vi "更新批次.vi"(8 "error in (no error)":errorcluster caption="错误输入", 11 "型号":string) -> (0 "error out":errorcluster caption="错误输出")   [LabVIEW 2018]
uses:
  <vilib>/addons/database/Connection.llb/DB Tools Open Connec (String).vi
  <vilib>/addons/database/Connection.llb/Conn Execute.vi
  <vilib>/addons/database/Recordset.llb/Rec Fetch Recordset Data (R).vi
  <vilib>/addons/database/Recordset.llb/Rec Destroy - Connection.vi
  <vilib>/addons/database/NI_Database_API.lvlib
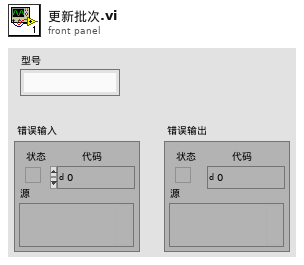
[diagram p1: front panel]
types:
  T1 = typedef "NI_Database_API.lvlib/Conn ObjectReference.ctl" = refnum<k1>
  T2 = typedef "NI_Database_API.lvlib/Rec ObjectReference.ctl" = refnum<k1>
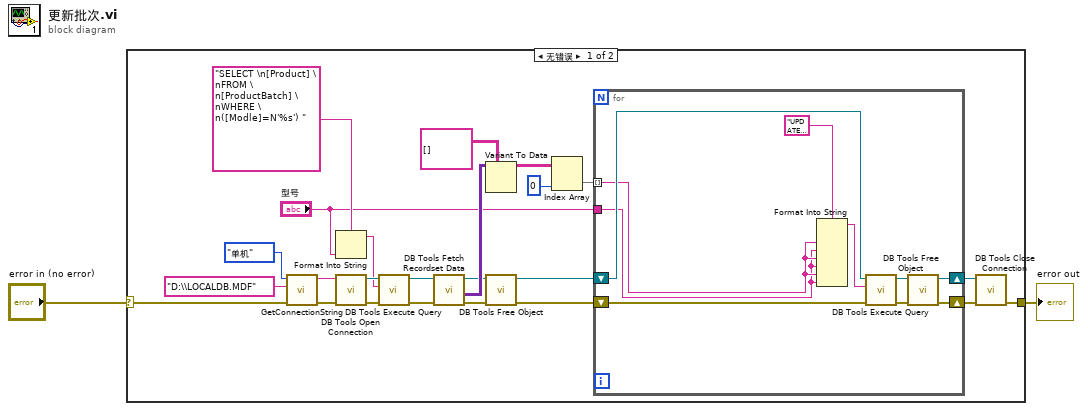
[diagram p0: block diagram]
diagram:
  n1 = case shown="无错误" "error in (no error)" {
    selector: "error in (no error)" -> [w6 w37]
    tunnel: [w19 w37] -> w1
    frame No Error {
      n2 = call "GetConnectionString.vi"("error in (no error)"=w6, "Database Name"="D:\\LOCALDB.MDF", "连接模式"=enum16{"单机", "联网"}."单机") -> ("error out"=w25:errorcluster, "连接字符串"=w24:string)  [unwired: 3 in]
      n3 = Format Into String(format string="SELECT \n[Product] \nFROM \n[ProductBatch] \nWHERE \n([Modle]=N'%s') " ("SQL query"), "型号") -> (resulting string=w4:string)  [unwired: 2 in, 1 out]
      n4 = call-poly <vilib>:"DB Tools Open Connection.vi"("error in (no error)"=w25, "connection information"=w24) -> ("error out"=w23:errorcluster, "connection reference"=w22:T1)  [unwired: 6 in]
      n5 = call-poly <vilib>:"DB Tools Execute Query.vi"("error in (no error)"=w23, "SQL query"=w4, "connection reference"=w22) -> ("error out"=w18:errorcluster, "recordset reference"=w17:T2)  [unwired: 5 in]
      n6 = call-poly <vilib>:"DB Tools Fetch Recordset Data.vi"("error in (no error)"=w18, "recordset reference"=w17) -> ("error out"=w11:errorcluster, "recordset data"=w16:variant[][], "recordset reference out"=w12:T2)  [unwired: 3 in]
      n7 = Variant To Data(type=string[][] [], Variant=w16) -> (data=w14:string[][])  [unwired: 1 in, 1 out]
      n8 = call-poly <vilib>:"DB Tools Free Object.vi"("error in (no error)"=w11, "recordset reference"=w12) -> ("error out"=w9:errorcluster, "connection reference"=w10:T1)  [unwired: 8 in]
      n9 = Index Array(array=w14, index (col)=0 ("禁用的索引 (列)")) -> (element=w8:string[])  [unwired: 1 in]
      n10 = for {
        shift-right: [w35] -> w20
        shift-left: w10 -> [w31]
        shift-right: [w36] -> w21
        shift-left: w9 -> [w30]
        tunnel: w8 -> [w28] mode=indexing
        tunnel: "型号" -> [w27]
        n11 = Format Into String(format string="UPDATE [ProductBatch] \nSET [Used]=(SELECT \n[Used] \nFROM \n[ProductBatch] \nWHERE \n[Product] =N'%s' AND \n[Modle]=N'%s')+(SELECT \n[Time] \nFROM \n[ProductBatch] \nWHERE \n[Product] =N'%s' AND \n[Modle]=N'%s') \nWHERE ([Product] =N'%s' \nAND [Modle]=N'%s') " ("格式字符串"), w28, w27, w28, w27, w28, w27) -> (resulting string=w29:string)  [unwired: 2 in, 1 out]
        n12 = call-poly <vilib>:"DB Tools Execute Query.vi"("error in (no error)"=w30, "SQL query"=w29, "connection reference"=w31) -> ("error out"=w32:errorcluster, "recordset reference"=w33:T2)  [unwired: 5 in]
        n13 = call-poly <vilib>:"DB Tools Free Object.vi"("error in (no error)"=w32, "recordset reference"=w33) -> ("error out"=w36:errorcluster, "connection reference"=w35:T1)  [unwired: 8 in]
      }
      n14 = call <vilib>:"DB Tools Close Connection.vi"("error in (no error)"=w21, "connection reference"=w20) -> ("error out"=w19:errorcluster)  [unwired: 5 in]
    }
    frame Error {
    }
  }
  "error out" <- w1
